vi "Get All Cluster Strings from Definition.vi"(4 "error in":errorcluster) -> (0 "error out":errorcluster, 3 "Cluster Strings":T1[](array[typedef]))   [LabVIEW 2025]
doc: "This VI generates an array of clusters that contain the name of each Cluster in the <i>Test Cluster Definition.xml</i> file, followed by all strings defined for each Cluster. This information is used to assert correct functioning of <b>Export Strings.vi</b>"
uses:
  Element Strings--cluster.ctl
  Cluster Definition--cluster.ctl
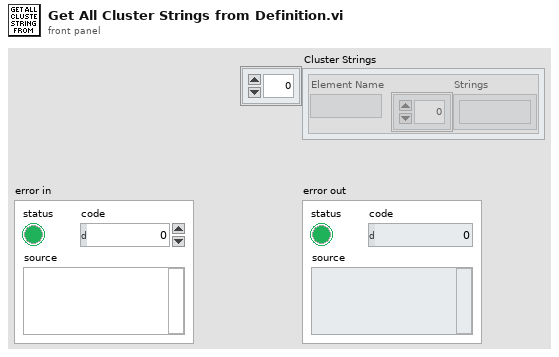
[diagram p1: front panel]
types:
  T1 = typedef "Element Strings--cluster.ctl" = cluster{"Element Name":string, "Strings":string[]}
  T2 = typedef "Cluster Definition--cluster.ctl" = cluster{"Name":string, "Description":string, "Numeric Indicators":cluster{"Labels":string[]}, "String Controls":cluster{"Labels":string[], "Default Values":string[]}, "Front Panel Labels":cluster{"Text":string[]}}
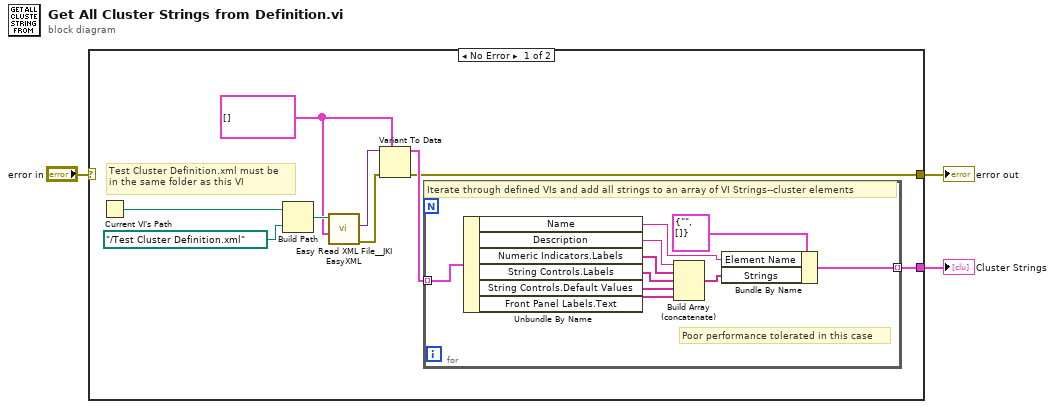
[diagram p0: block diagram]
diagram:
  n1 = case shown="No Error" "error in" {
    selector: "error in" -> [_ w23]
    tunnel: [w4 _] -> w3
    tunnel: [w5 w23] -> w1
    frame No Error {
      w7 = T2[] [] ("Array")
      # "Test Cluster Definition.xml must be\nin the same folder as this VI"
      n2 = Current VI's Path() -> (path=w12:path)
      n3 = Build Path(base path=w12, name or relative path=path "../Test Cluster Definition.xml") -> (appended path=w10:path)
      n4 = call <vilib>:"Easy Read XML File__JKI EasyXML.vi"("LabVIEW Data (Type)"=w7, "XML File Path"=w10) -> ("error out"=w8:errorcluster, "LabVIEW Data"=w9:variant)  [unwired: 7 in, 1 out]
      n5 = Variant To Data(error in=w8, type=w7, Variant=w9) -> (data=w6:T2[], error out=w5:errorcluster)
      n6 = for {
        tunnel: w6 -> [w22] mode=indexing
        tunnel: [w13] -> w4 mode=indexing
        # "Poor performance tolerated in this case"
        # "Iterate through defined VIs and add all strings to an array of VI Strings--cluster elements"
        n7 = Unbundle By Name(w22) -> ("Name"=w16:string, "Description"=w21:string, "Numeric Indicators.Labels"=w20:string[], "String Controls.Labels"=w19:string[], "String Controls.Default Values"=w18:string[], "Front Panel Labels.Text"=w17:string[])
        n8 = Build Array (concatenate)(w21, w20, w19, w18, w17) -> (w15:string[])
        n9 = Bundle By Name(cluster=T1 {"Element Name"="", "Strings"=[]} ("VI Strings"), "Element Name"=w16, "Strings"=w15) -> (w13:T1)
      }
    }
    frame Error {
      # "Pass error without  further action"
    }
  }
  "Cluster Strings" <- w3
  "error out" <- w1
